vi "Write Cooler.vi"(10 "Cooler":refnum<class "Message Enqueuer.lvclass">, 11 "Cooler UI with Events in":refnum<class "Cooler UI with Events.lvclass">=refnum) -> (3 "Cooler UI with Events out":refnum<class "Cooler UI with Events.lvclass">)   [LabVIEW 2012, in "Cooler UI.lvlib" / "Cooler UI with Events.lvclass"]
uses:
  Cooler UI with Events.lvclass
  <vilib>/ActorFramework/Message Enqueuer/Message Enqueuer.lvclass
  Cooler UI with Events.lvclass/Cooler UI with Events.ctl
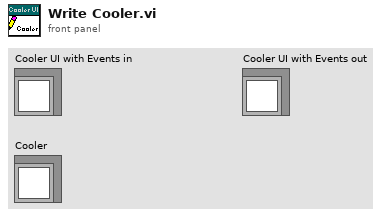
[diagram p1: front panel]
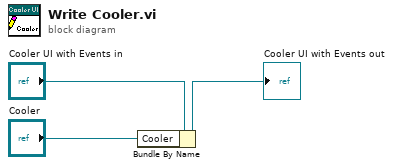
[diagram p0: block diagram]
diagram:
  n1 = Bundle By Name(cluster="Cooler UI with Events in", "Cooler"="Cooler") -> (→"Cooler UI with Events out":refnum<class "Cooler UI with Events.lvclass">)
